vi "Interpret Joysticks.vi"(10 "Joystick Controls":T6={"Driver Left Joystick X"=0.0, "Driver Left Joystick Y"=0.0, "Driver A Button"=FALSE, "Driver B Button"=FALSE, "Driver X Button"=FALSE, "Driver Y Button"=FALSE, "Driver Left Bumper"=FALSE, "Driver Right Bumper"=FALSE, "Driver View Button"=FALSE, "Driver Menu Button"=FALSE, "Driver Left Joystick Press"=FALSE, "Driver Right Joystick Press"=FALSE, "Driver Left Trigger"=0.0, "Driver Right Joystick X"=0.0, "Driver Right Joystick Y"=0.0, "Driver Right Trigger"=0.0, "Operator Left Joystick X"=0.0, "Operator Left Joystick Y"=0.0, "Operator A Button"=FALSE, "Operator B Button"=FALSE, "Operator X Button"=FALSE, "Operator Y Button"=FALSE, "Operator Left Bumper"=FALSE, "Operator Right Bumper"=FALSE, "Operator View Button"=FALSE, "Operator Menu Button"=FALSE, "Operator Left Joystick Press"=FALSE, "Operator Right Joystick Press"=FALSE, "Operator Left Trigger"=0.0, "Operator Right Joystick X"=0.0, "Operator Right Joystick Y"=0.0, "Operator Right Trigger"=0.0, "Driver D-Pad"=-1, "Operator D-Pad"=-1}) -> (0 "Climb Outputs":T2, 1 "Teleop Hatch and Cargo":T3, 2 "4bar output":T5 {"Control Mode" items=["PercentOutput"=0, "Position"=1, "Velocity"=2, "Current"=3, "Follower"=5, "MotionProfile"=6, "MotionMagic"=7, "MotionProfileArc"=10, "Disabled"=15]}, 3 "Drive Motor Values":cluster{"Left Motor":dbl, "Right Motor":dbl})   [LabVIEW 2018]
uses:
  Joystick Controls.ctl
  <vilib>/Rock Robotics/WPI/ThirdParty/Phoenix-LabVIEW/Motor Controller/Controls/CTRE_Phoenix_MotorControl_ControlMode.ctl
  <vilib>/Rock Robotics/WPI/Solenoid/WPI_SolenoidValue.ctl
  Robot Global Data.vi
panel:
  out "Rear Climb Output":T1
  out "Front Climb Output":T1
  # "NOT DONE"
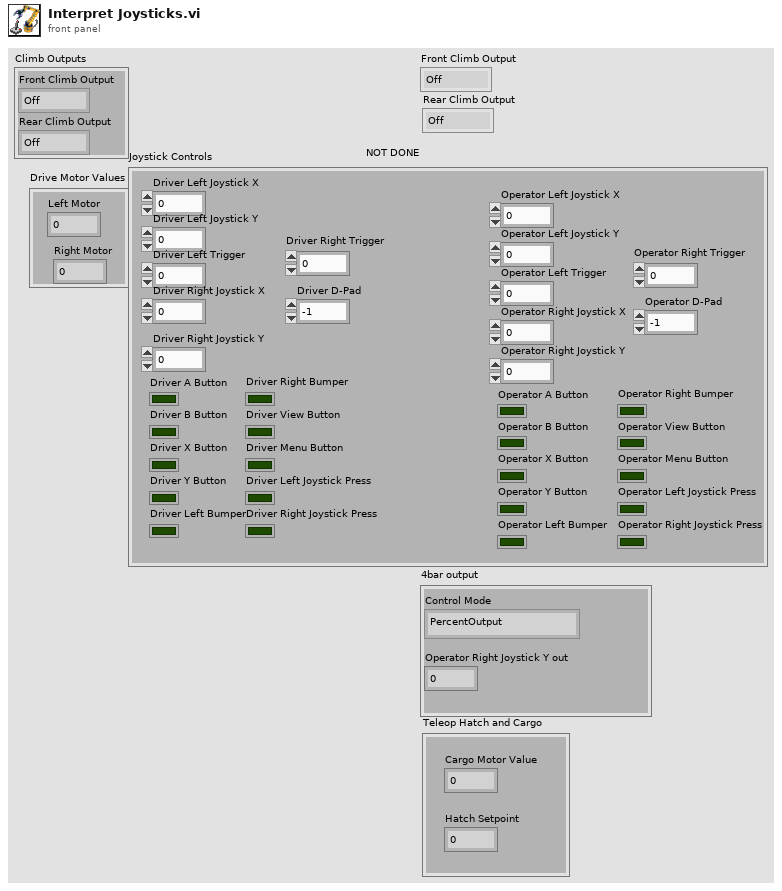
[diagram p1: front panel]
types:
  T1 = typedef "WPI_SolenoidValue.ctl" = enum16{"Off", "On", "Forward", "Reverse"}
  T2 = cluster{"Front Climb Output":T1, "Rear Climb Output":T1}
  T3 = cluster{"Cargo Motor Value":dbl, "Hatch Setpoint":dbl}
  T4 = typedef "CTRE_Phoenix_MotorControl_ControlMode.ctl" = u16
  T5 = cluster{"Control Mode":T4, "Operator Right Joystick Y out":dbl}
  T6 = typedef "Joystick Controls.ctl" = cluster{"Driver Left Joystick X":dbl, "Driver Left Joystick Y":dbl, "Driver A Button":bool, "Driver B Button":bool, "Driver X Button":bool, "Driver Y Button":bool, "Driver Left Bumper":bool, "Driver Right Bumper":bool, "Driver View Button":bool, "Driver Menu Button":bool, "Driver Left Joystick Press":bool, "Driver Right Joystick Press":bool, "Driver Left Trigger":dbl, "Driver Right Joystick X":dbl, "Driver Right Joystick Y":dbl, "Driver Right Trigger":dbl, "Operator Left Joystick X":dbl, "Operator Left Joystick Y":dbl, "Operator A Button":bool, "Operator B Button":bool, "Operator X Button":bool, "Operator Y Button":bool, "Operator Left Bumper":bool, "Operator Right Bumper":bool, "Operator View Button":bool, "Operator Menu Button":bool, "Operator Left Joystick Press":bool, "Operator Right Joystick Press":bool, "Operator Left Trigger":dbl, "Operator Right Joystick X":dbl, "Operator Right Joystick Y":dbl, "Operator Right Trigger":dbl, "Driver D-Pad":i16, "Operator D-Pad":i16}
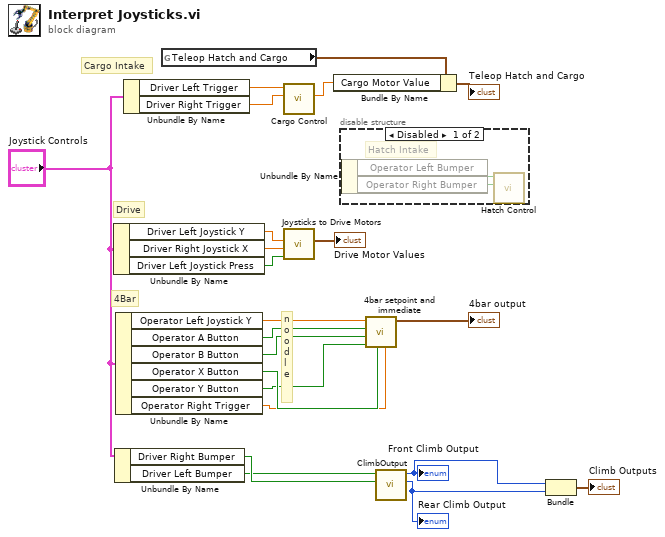
[diagram p0: block diagram]
diagram:
  # "n\no\no\nd\nl\ne"
  # "Cargo Intake"
  # "4Bar"
  # "Drive"
  n1 = Unbundle By Name("Joystick Controls") -> ("Driver Left Joystick Y"=w20:dbl, "Driver Right Joystick X"=w21:dbl, "Driver Left Joystick Press"=w22:bool)
  n2 = Unbundle By Name("Joystick Controls") -> ("Driver Right Bumper"=w5:bool, "Driver Left Bumper"=w4:bool)
  n3 = Unbundle By Name("Joystick Controls") -> ("Operator Left Joystick Y"=w18:dbl, "Operator A Button"=w17:bool, "Operator B Button"=w16:bool, "Operator X Button"=w15:bool, "Operator Y Button"=w14:bool, "Operator Right Trigger"=w7:dbl)
  n4 = Unbundle By Name("Joystick Controls") -> ("Driver Left Trigger"=w12:dbl, "Driver Right Trigger"=w11:dbl)
  n5 = global read "Robot Global Data.vi" "Teleop Hatch and Cargo"() -> (w9:T3)
  n6 = call "Cargo Control.vi"("Operator Right Trigger"=w11, "Operator Left Trigger"=w12) -> ("Numeric"=w10:dbl)  [unwired: 9 in]
  n7 = call "Joysticks to Drive Motors.vi"("Boost?"=w22, "Turn"=w21, "Throttle"=w20) -> ("Drive Motor Values"=→"Drive Motor Values":cluster{"Left Motor":dbl, "Right Motor":dbl})  [unwired: 8 in]
  n8 = Bundle By Name(cluster=w9, "Cargo Motor Value"=w10) -> (→"Teleop Hatch and Cargo":T3)
  n9 = disable-structure shown="Disabled" {
    frame Disabled {
      # "Hatch Intake"
      n10 = Unbundle By Name() -> ("Operator Left Bumper"=w24:bool, "Operator Right Bumper"=w23:bool)  [unwired: 1 in]
      n11 = call "Hatch Control.vi"("Driver Right Bumper"=w23, "Driver Left Bumper"=w24) -> ()  [unwired: 9 in, 1 out]
    }
    frame Enabled {
    }
  }
  n12 = call "4bar setpoint and immediate.vi"("Cargo Ship for Cargo"=w7, "Operator X Button"=w15, "Operator Y Button"=w14, "Operator B Button"=w16, "Operator A Button"=w17, "Operator Right Joystick Y in"=w18) -> ("Output"=→"4bar output":cluster{"Control Mode":T4, "Output":dbl})  [unwired: 5 in]
  n13 = call "ClimbOutput.vi"("Driver Right Bumper"=w5, "Driver Left Bumper"=w4) -> ("Rear Climb Output"=w2:T1, "Front Climb Output"=w3:T1)  [unwired: 8 in]
  "Front Climb Output" <- w3
  "Rear Climb Output" <- w2
  n14 = Bundle("Front Climb Output"=w3, "Rear Climb Output"=w2) -> (→"Climb Outputs":T2)  [unwired: 1 in]
